vi "Read Type.vi"(8 "Error In":errorcluster, 11 "String In":refnum<class "String.lvclass">) -> (0 "Error Out":errorcluster, 2 "Type":T1=enum."String", 3 "String Out":refnum<class "String.lvclass">)   [LabVIEW 2018, in "Toolkit.lvlib" / "Data.lvlib" / "String.lvclass"]
doc: "Gets the Mustache data type of an object. This is primarily used internally or when building custom compilers. This is more robust than using strings in case structures with the Get LV Class Name function, which is not available in older versions of LabVIEW.\n\n<B>String In/Out</B> - Represents a Mustache string value.\n\n<B>Type</B> - Indicates the data type as an enum."
uses:
  String.lvclass
  Type Defintions/Types.ctl
  Data.lvlib
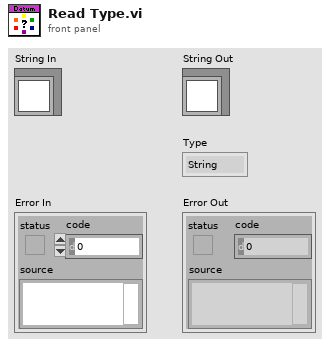
[diagram p1: front panel]
types:
  T1 = typedef "Toolkit.lvlib/Data.lvlib/Types.ctl" = enum16{"Array", "Boolean", "Function", "Map", "Null", "Pair", "Path", "String", "Unknown"}
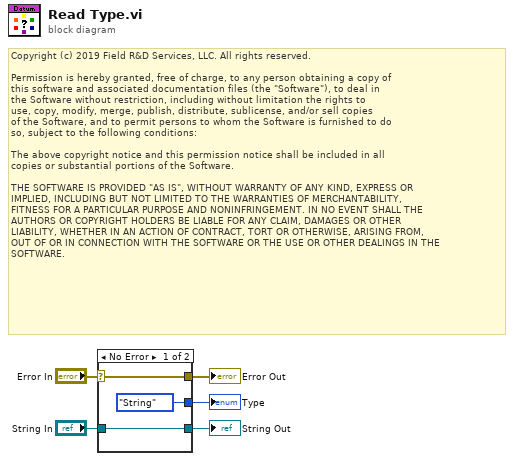
[diagram p0: block diagram]
diagram:
  # "Copyright (c) 2019 Field R&D Services, LLC. All rights reserved.\n\nPermission is hereby granted, free of charge, to any person obtaining a copy of\nthis software and associated documentation files (the \"Software\"), to deal in\nthe Software without restriction, including without limitation the rights to\nuse, copy, modify, merge, publish, distribute, sublicense, and/or sell copies\nof the Software, and to permit persons to whom the Software is furnished to do\nso, subject to the following conditions:\n\nThe above copyright notice and this permission notice shall be included in all\ncopies or substantial portions of the Software.\n\nTHE SOFTWARE IS PROVIDED \"AS IS\", WITHOUT WARRANTY OF ANY KIND, EXPRESS OR\nIMPLIED, INCLUDING BUT NOT LIMITED TO THE WARRANTIES OF MERCHANTABILITY,\nFITNESS FOR A PARTICULAR PURPOSE AND NONINFRINGEMENT. IN NO EVENT SHALL THE\nAUTHORS OR COPYRIGHT HOLDERS BE LIABLE FOR ANY CLAIM, DAMAGES OR OTHER\nLIABILITY, WHETHER IN AN ACTION OF CONTRACT, TORT OR OTHERWISE, ARISING FROM,\nOUT OF OR IN CONNECTION WITH THE SOFTWARE OR THE USE OR OTHER DEALINGS IN THE\nSOFTWARE."
  n1 = case shown="No Error" "Error In" {
    selector: "Error In" -> [w8 w9]
    tunnel: [w8 w9] -> w4
    tunnel: "String In" -> [w7 w10]
    tunnel: [w7 w10] -> w2
    tunnel: [Types."String" ("Type") _] -> w1
    frame No Error {
    }
    frame Error {
    }
  }
  "Error Out" <- w4
  "String Out" <- w2
  "Type" <- w1
